vi "Test Compare I32.vi"   [LabVIEW 2020, in "Caraya Test 2.lvlib"]
uses:
  Caraya Test 2.lvlib
  <vilib>/addons/_JKI Toolkits/Caraya/classes/Assert/Assert Equal Value_Variant.vi
  <vilib>/addons/_JKI Toolkits/Caraya/classes/Test/Test.lvclass
  <vilib>/addons/_JKI Toolkits/Caraya/classes/Assert/Assert.lvclass
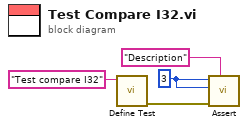
[diagram p0: block diagram]
diagram:
  w2 = 3
  n1 = call <vilib>:"Define Test.vi"("Label (VI Title)"="Test compare I32" ("Description")) -> ("error out"=w4:errorcluster)  [unwired: 10 in]
  n2 = call-poly <vilib>:"Assert.vi"("Label"="Description" ("Description"), "error in (no error)"=w4, "Y"=w2, "X"=w2) -> ()  [unwired: 7 in, 1 out]
